vi "Thermometer.vi"(7 "에러 입력(에러 없음)":errorcluster, 9 "온도 스케일":bool) -> (0 "에러 출력":errorcluster, 2 "온도":dbl(slide) scale=0.0..100.0 scale format="%.1f")   [LabVIEW 2010]
panel:
  # "섭씨\n\n화씨"
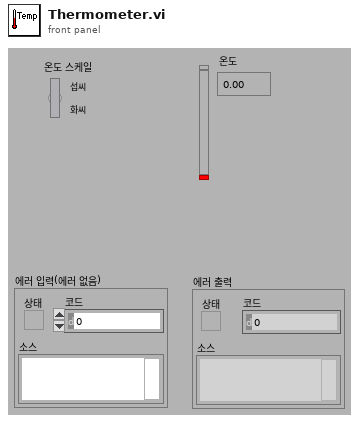
[diagram p1: front panel]
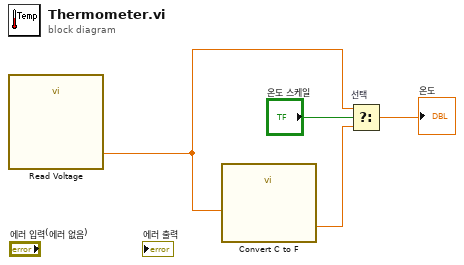
[diagram p0: block diagram]
diagram:
  n1 = call "Read Voltage.vi"() -> ("전압"=w1:dbl)  [unwired: 6 in, 1 out]
  n2 = call "Convert C to F.vi"("섭씨"=w1) -> ("화씨"=w2:dbl)
  n3 = Select "선택"(t=w1, s="온도 스케일", f=w2) -> (s? t:f=→"온도":dbl)
